vi "SWERVE_DRIVE_MODULE_OPEN.vi"(3 "NameSuffix":string="0", 4 "RadiansPerCount":dbl=1.0, 5 "Drive PWM Channel":T2, 6 "DistancePerCount":dbl=1.0, 7 "Swerve PWM Channel":T2, 8 "Swerve B Channel":T1, 9 "Swerver A Channel":T1, 10 "Drive B Channel":T1, 11 "Drive A channel":T1) -> ()   [LabVIEW 2019]
uses:
  <vilib>/Rock Robotics/SystemInterfaces/DIO/FPGA_DIOChannel.ctl
  <vilib>/Rock Robotics/SystemInterfaces/DIO/FPGA_DIOPWMChannel.ctl
  <vilib>/Rock Robotics/WPI/MotorControl/WPI_MotorControlOpen SPARK.vi
  <vilib>/Rock Robotics/WPI/Counter/WPI_CounterDigitalInputToDigitalSource.vi
  <vilib>/Rock Robotics/WPI/SafetyOutput/WPI_SafetyOutputConfigMenu.ctl
  <vilib>/Rock Robotics/WPI/Encoder/WPI_EncoderType.ctl
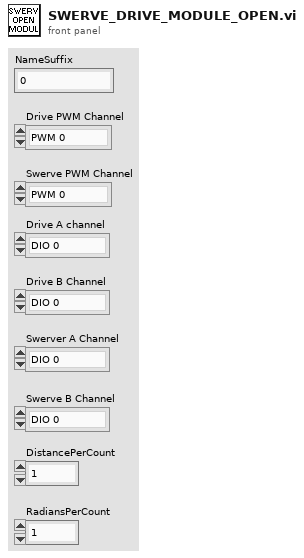
[diagram p1: front panel]
types:
  T1 = typedef "FPGA_DIOChannel.ctl" = enum8{"DIO 0", "DIO 1", "DIO 2", "DIO 3", "DIO 4", "DIO 5", "DIO 6", "DIO 7", "DIO 8", "DIO 9", "DIO MXP 0", "DIO MXP 1", "DIO MXP 2", "DIO MXP 3", "DIO MXP 4", "DIO MXP 5", "DIO MXP 6", "DIO MXP 7", "DIO MXP 8", "DIO MXP 9", "DIO MXP 10", "DIO MXP 11", "DIO MXP 12", "DIO MXP 13", "DIO MXP 14", "DIO MXP 15", "SPI Port CS1", "SPI Port CS2", "SPI Port CS3", "SPI Port MISO", "SPI Port MOSI", "Invalid"}
  T2 = typedef "FPGA_DIOPWMChannel.ctl" = enum8{"PWM 0", "PWM 1", "PWM 2", "PWM 3", "PWM 4", "PWM 5", "PWM 6", "PWM 7", "PWM 8", "PWM 9", "PWM MXP 0", "PWM MXP 1", "PWM MXP 2", "PWM MXP 3", "PWM MXP 4", "PWM MXP 5", "PWM MXP 6", "PWM MXP 7", "PWM MXP 8", "PWM MXP 9", "Invalid"}
  T3 = typedef "WPI_EncoderType.ctl" = enum16{"1x", "2x", "4x"}
  T4 = typedef "WPI_SafetyOutputConfigMenu.ctl" = enum16{"Enable", "Disable"}
  T5 = typedef "WPI_MotorControlDeviceRef.ctl" = cluster{"DeviceStatus":errorcluster, "Type":T6, "PWM":cluster{"PWM Channel":T2, "DeadBand":T7}, "CAN":cluster{"Device Number":u8, "SetOutput VI Ref":variant, "GetOutput VI Ref":variant, "Enable VI Ref":variant, "Disable VI Ref":variant, "Data":variant}, "Invert":bool, "DIO PWM":cluster{"PWM \"Enable\" Channel":T2, "DIOChannel":T1, "PWM Rate":dbl}}
  T6 = typedef "WPI_MotorControlType.ctl" = enum16{"PWM", "CAN", "DIO PWM"}
  T7 = typedef "WPI_PWMDeadband.ctl" = cluster{"Name":string, "maxPositivePwm":i32, "minPositivePwm":i32, "centerPwm":i32, "maxNegativePwm":i32, "minNegativePwm":i32, "angularRange":u16}
  T8 = typedef "WPI_DigitalInputDevRef.ctl" = cluster{"DevStatus":errorcluster, "DIO Channel":T1}
  T9 = typedef "FPGA_CounterEncoderSourceConvertionLVSourceType.ctl" = cluster{"DevStatus":errorcluster, "AnalogTriggerMode?":bool, "DigitalMode":cluster{"DIO Channel":T10}, "AnalogTriggerMode":cluster{"AnalogTriggerIndex":T11, "OutputType":T12}}
  T10 = typedef "FPGA_DIODigitalSourceChannel.ctl" = enum8{"DIO 0", "DIO 1", "DIO 2", "DIO 3", "DIO 4", "DIO 5", "DIO 6", "DIO 7", "DIO 8", "DIO 9", "DIO MXP 0", "DIO MXP 1", "DIO MXP 2", "DIO MXP 3", "DIO MXP 4", "DIO MXP 5", "DIO MXP 6", "DIO MXP 7", "DIO MXP 8", "DIO MXP 9", "DIO MXP 10", "DIO MXP 11", "DIO MXP 12", "DIO MXP 13", "DIO MXP 14", "DIO MXP 15", "SPI Port CS1", "SPI Port CS2", "SPI Port CS3", "SPI Port MISO", "SPI Port MOSI", "Disabled"}
  T11 = typedef "FPGA_AnalogTriggerIndex.ctl" = enum8{"Trig 0", "Trig 1", "Trig 2", "Trig 3", "Trig 4", "Trig 5", "Trig 6", "Trig 7", "Invalid"}
  T12 = typedef "FPGA_AnalogTriggerOutType.ctl" = enum16{"InWindow", "TriggerState", "Rising", "Falling"}
  T13 = typedef "WPI_EncoderDevRef.ctl" = cluster{"DevStatus":errorcluster, "EncoderIndex":T14, "CounterIndex":T15, "DistancePerCount":dbl, "Decoding Type":T3}
  T14 = typedef "FPGA_EncoderIdx.ctl" = enum8{"Enc 0", "Enc 1", "Enc 2", "Enc 3", "Enc 4", "Enc 5", "Enc 6", "Enc 7", "Invalid"}
  T15 = typedef "FPGA_CounterCtrSystemIndex.ctl" = enum8{"Ctr 0", "Ctr 1", "Ctr 2", "Ctr 3", "Ctr 4", "Ctr 5", "Ctr 6", "Ctr 7", "Invalid"}
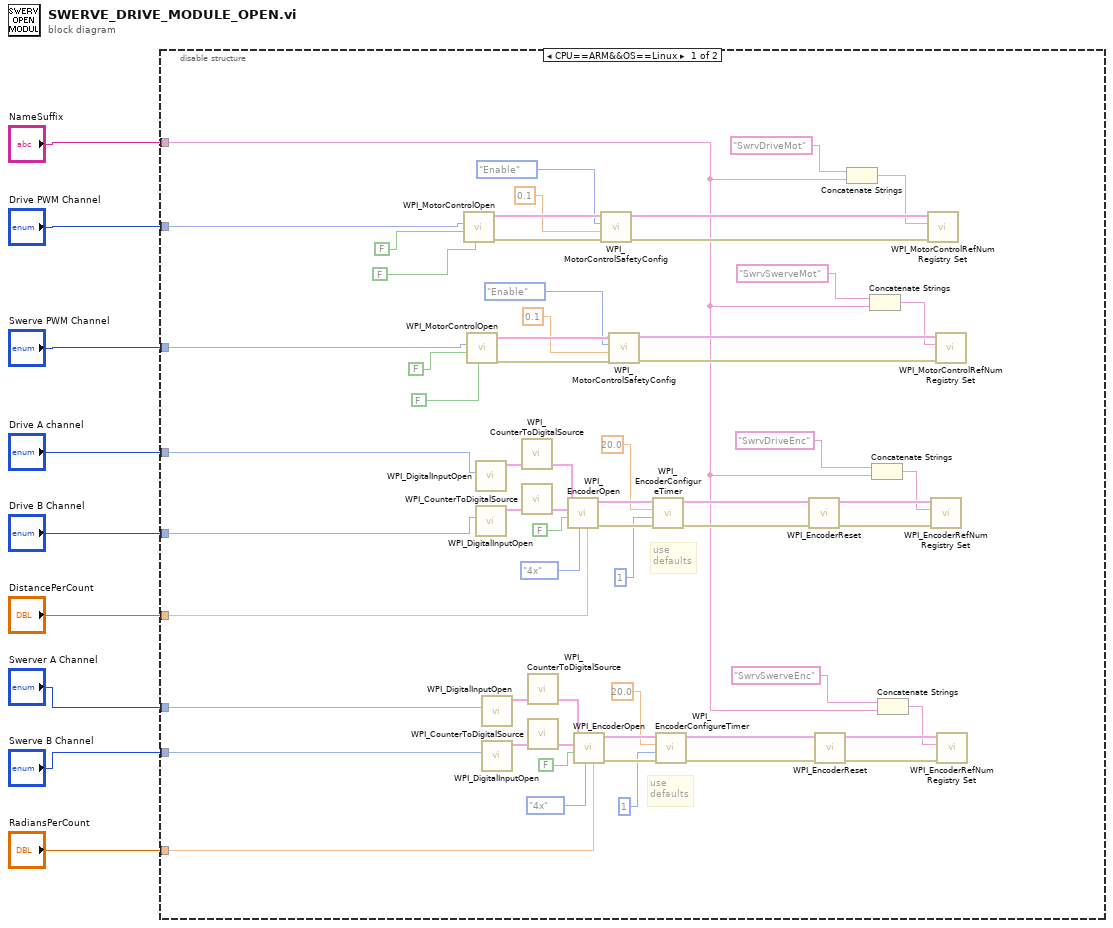
[diagram p0: block diagram]
diagram:
  n1 = disable-structure shown="CPU==ARM&&OS==Linux" {
    disable-tunnel: "NameSuffix" -> [w27 _]
    disable-tunnel: "Swerve B Channel" -> [w35 _]
    disable-tunnel: "Swerver A Channel" -> [w34 _]
    disable-tunnel: "RadiansPerCount" -> [w33 _]
    disable-tunnel: "Drive B Channel" -> [w20 _]
    disable-tunnel: "Drive A channel" -> [w19 _]
    disable-tunnel: "DistancePerCount" -> [w18 _]
    disable-tunnel: "Swerve PWM Channel" -> [w13 _]
    disable-tunnel: "Drive PWM Channel" -> [w10 _]
    frame condition #0 {
      # "use\ndefaults"
      # "use\ndefaults"
      n2 = call-poly <vilib>:"WPI_MotorControlOpen.vi"("Invert"=FALSE, "Eliminate Deadband"=FALSE, "PWM Channel"=w10) -> ("error out"=w65:errorcluster, "MotorControlDeviceRef"=w66:T5)  [unwired: 7 in]
      n3 = call-poly <vilib>:"WPI_MotorControlOpen.vi"("Invert"=FALSE, "Eliminate Deadband"=FALSE, "PWM Channel"=w13) -> ("error out"=w59:errorcluster, "MotorControlDeviceRef"=w60:T5)  [unwired: 7 in]
      n4 = call <vilib>:"WPI_DigitalInputOpen.vi"("DIO Channel"=w19) -> ("DigitalInputDevRef"=w68:T8)  [unwired: 1 in, 9 out]
      n5 = call <vilib>:"WPI_DigitalInputOpen.vi"("DIO Channel"=w20) -> ("DigitalInputDevRef"=w69:T8)  [unwired: 1 in, 9 out]
      n6 = call <vilib>:"WPI_DigitalInputOpen.vi"("DIO Channel"=w34) -> ("DigitalInputDevRef"=w47:T8)  [unwired: 1 in, 9 out]
      n7 = call <vilib>:"WPI_DigitalInputOpen.vi"("DIO Channel"=w35) -> ("DigitalInputDevRef"=w48:T8)  [unwired: 1 in, 9 out]
      n8 = call-poly <vilib>:"WPI_CounterToDigitalSource.vi"("DigitalInputDevRef"=w68) -> ("Digital Source"=w67:T9)  [unwired: 6 out]
      n9 = call-poly <vilib>:"WPI_CounterToDigitalSource.vi"("DigitalInputDevRef"=w69) -> ("Digital Source"=w70:T9)  [unwired: 6 out]
      n10 = call-poly <vilib>:"WPI_CounterToDigitalSource.vi"("DigitalInputDevRef"=w47) -> ("Digital Source"=w46:T9)  [unwired: 6 out]
      n11 = call-poly <vilib>:"WPI_CounterToDigitalSource.vi"("DigitalInputDevRef"=w48) -> ("Digital Source"=w49:T9)  [unwired: 6 out]
      n12 = call <vilib>:"WPI_EncoderOpen.vi"("DistancePerCount"=w18, "Decoding Type"=WPI_EncoderType."4x", "Invert Direction (False)"=FALSE, "BSource"=w70, "ASource"=w67) -> ("error out"=w57:errorcluster, "EncoderDevRef"=w58:T13)  [unwired: 3 in, 2 out]
      n13 = call <vilib>:"WPI_EncoderOpen.vi"("DistancePerCount"=w33, "Decoding Type"=WPI_EncoderType."4x", "Invert Direction (False)"=FALSE, "BSource"=w49, "ASource"=w46) -> ("error out"=w44:errorcluster, "EncoderDevRef"=w45:T13)  [unwired: 3 in, 2 out]
      n14 = call <vilib>:"WPI_MotorControlSafetyConfig.vi"("error in (no error)"=w65, "timeout (s)"=0.1, "mode"=WPI_SafetyOutputConfigMenu."Enable", "MotorControlDevRef"=w66) -> ("error out"=w63:errorcluster, "MotorControlDevRef"=w64:T5)  [unwired: 6 in]
      n15 = call <vilib>:"WPI_MotorControlSafetyConfig.vi"("error in (no error)"=w59, "timeout (s)"=0.1, "mode"=WPI_SafetyOutputConfigMenu."Enable", "MotorControlDevRef"=w60) -> ("error out"=w61:errorcluster, "MotorControlDevRef"=w62:T5)  [unwired: 6 in]
      n16 = call <vilib>:"WPI_EncoderConfigureTimer.vi"("error in (no error)"=w57, "Number Samples to Average"=u8 1, "Minimum Rate"=20.0, "EncoderDevRef"=w58) -> ("error out"=w56:errorcluster, "EncoderDevRef"=w54:T13)  [unwired: 6 in]
      n17 = call <vilib>:"WPI_EncoderConfigureTimer.vi"("error in (no error)"=w44, "Number Samples to Average"=u8 1, "Minimum Rate"=20.0, "EncoderDevRef"=w45) -> ("error out"=w43:errorcluster, "EncoderDevRef"=w41:T13)  [unwired: 6 in]
      n18 = call <vilib>:"WPI_EncoderReset.vi"("error in (no error)"=w56, "EncoderDevRef"=w54) -> ("error out"=w55:errorcluster, "EncoderDevRef"=w53:T13)  [unwired: 8 in]
      n19 = call <vilib>:"WPI_EncoderReset.vi"("error in (no error)"=w43, "EncoderDevRef"=w41) -> ("error out"=w42:errorcluster, "EncoderDevRef"=w40:T13)  [unwired: 8 in]
      n20 = Concatenate Strings("SwrvDriveMot" ("refnum name"), w27) -> (w52:string)
      n21 = Concatenate Strings("SwrvSwerveMot" ("refnum name"), w27) -> (w51:string)
      n22 = Concatenate Strings("SwrvDriveEnc" ("refnum name"), w27) -> (w50:string)
      n23 = Concatenate Strings("SwrvSwerveEnc" ("refnum name"), w27) -> (w39:string)
      n24 = call <vilib>:"WPI_MotorControlRefNum Registry Set.vi"("error in (no error)"=w63, "refnum name"=w52, "MotorControlDevRef"=w64) -> ()  [unwired: 7 in, 2 out]
      n25 = call <vilib>:"WPI_EncoderRefNum Registry Set.vi"("error in (no error)"=w55, "refnum name"=w50, "EncoderDevRef"=w53) -> ()  [unwired: 7 in, 2 out]
      n26 = call <vilib>:"WPI_MotorControlRefNum Registry Set.vi"("error in (no error)"=w61, "refnum name"=w51, "MotorControlDevRef"=w62) -> ()  [unwired: 7 in, 2 out]
      n27 = call <vilib>:"WPI_EncoderRefNum Registry Set.vi"("error in (no error)"=w42, "refnum name"=w39, "EncoderDevRef"=w40) -> ()  [unwired: 7 in, 2 out]
    }
    frame condition #1 (active) {
      # "DO NOTHING ON WINDOWS...."
    }
  }
